vi "Get Selected XNET Channels.vi"(4 "Delete Olds?":bool, 6 "Add Info?":bool, 8 "error in (no error)":errorcluster, 9 "Node Ptr":u64 format="%.0x", 10 "XNET Cluster":refnum<k21>, 11 "Tree In":refnum<vi>) -> (0 "error out":errorcluster, 2 "XNET Signal Names":refnum<k21>[](array[refnum]), 3 "Tree Out":refnum<vi>)   [LabVIEW 2023, in "Protection and Counter Addon System Explorer.lvlib"]
uses:
  Protection and Counter Addon System Explorer.lvlib
  <resource>/objmgr/xnet.rc
  <vilib>/NI VeriStand/Custom Device API/Custom Device API.lvlib
panel:
  # "OUTPUTS"
  # "INPUTS"
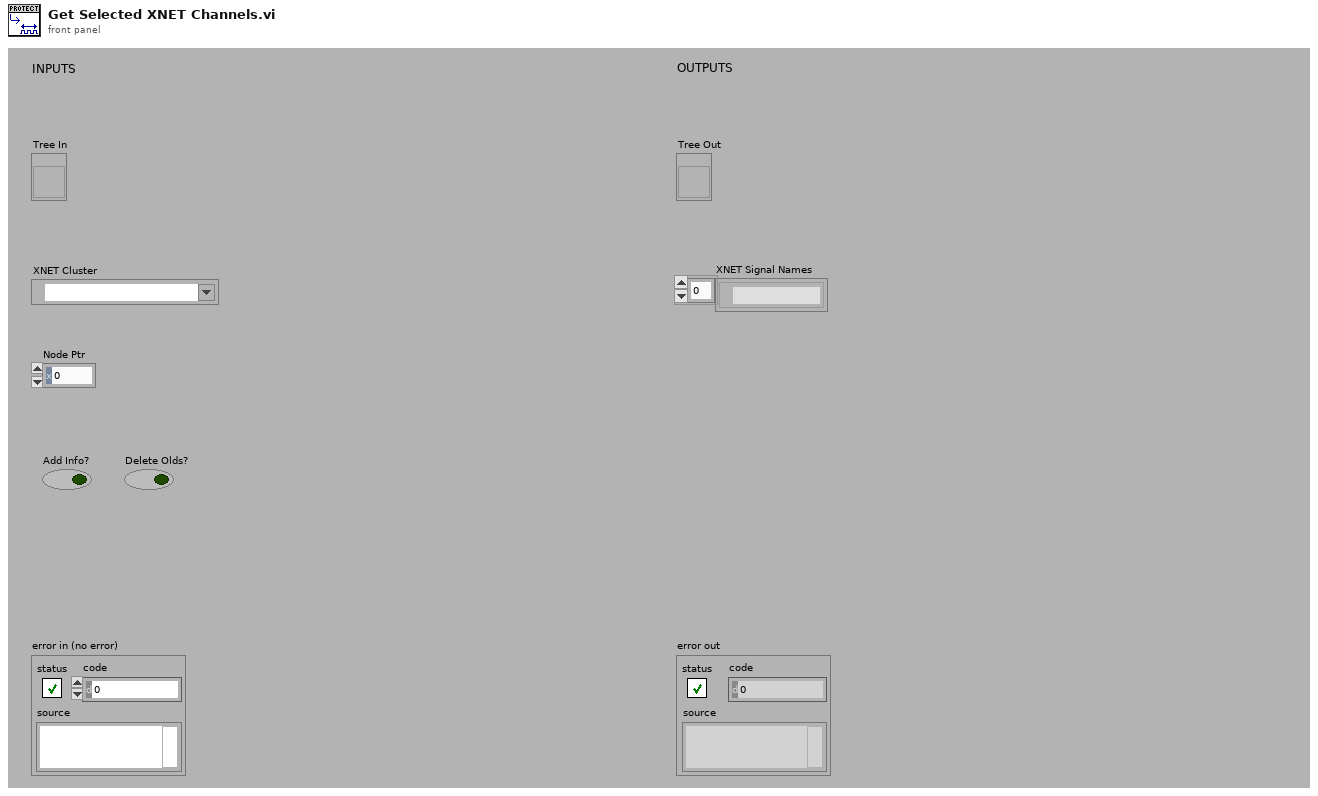
[diagram p1: front panel]
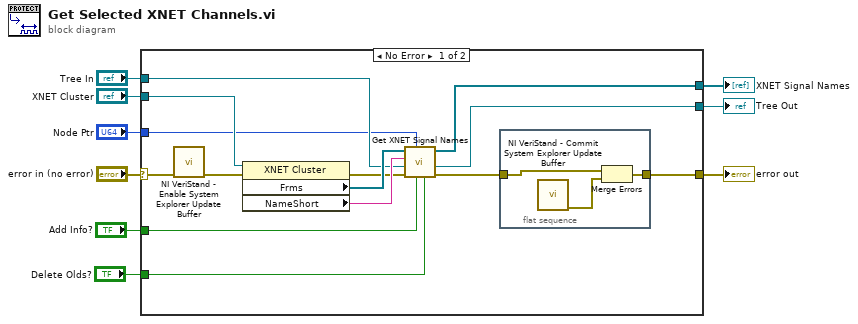
[diagram p0: block diagram]
diagram:
  n1 = case shown="No Error" "error in (no error)" {
    selector: "error in (no error)" -> [w16 w28]
    tunnel: [w14 w28] -> w8
    tunnel: "XNET Cluster" -> [w23 _]
    tunnel: [w18 _] -> w6
    tunnel: "Tree In" -> [w17 w27]
    tunnel: [w20 w27] -> w4
    tunnel: "Node Ptr" -> [w12 _]
    tunnel: "Add Info?" -> [w13 _]
    tunnel: "Delete Olds?" -> [w10 _]
    frame No Error {
      n2 = call <vilib>:"NI VeriStand - Enable System Explorer Update Buffer.vi"("error in (no error)"=w16) -> ("error out"=w11:errorcluster)  [unwired: 10 in]
      n3 = property class="XNET Cluster"(reference=w23, error in=w11) -> (error out=w19:errorcluster, "Frms"=w22:refnum<k21>[], "NameShort"=w21:string)  [unwired: 1 out]
      n4 = call "Get XNET Signal Names.vi"("Delete Olds?"=w10, "Add Info?"=w13, "Parent Ref in"=w12, "error in"=w19, "Tree In"=w17, "Parent"=w21, "Frms"=w22) -> ("error out"=w15:errorcluster, "Tree Out"=w20:refnum<vi>, "XNET Signal Names"=w18:refnum<k21>[])  [unwired: 2 in]
      n5 = flat-sequence {
        tunnel: w15 -> [w25]
        tunnel: [w24] -> w14
        frame #0 {
          n6 = call <vilib>:"NI VeriStand - Commit System Explorer Update Buffer.vi"() -> ("error out"=w26:errorcluster)  [unwired: 11 in]
          n7 = Merge Errors(w25, w26) -> (w24:errorcluster)
        }
      }
    }
    frame Error {
    }
  }
  "error out" <- w8
  "XNET Signal Names" <- w6
  "Tree Out" <- w4
